vi "Convert Pressure (inHg) to Altitude (ft).vi"(10 "Altimeter Setting (inHg)":dbl=29.9213, 11 "Pressure (inHg)":dbl) -> (3 "Altitude (ft)":dbl)   [LabVIEW 2020, in "LPS Barometric Pressure Sensor.lvclass"]
doc: "Converts pressure in mbar to altitude in meters, using 1976 US Standard Atmosphere model (only applicable up to height of 11km/36,000ft). If altimeter setting (QNH, barometric pressure adjusted to sea level) is given, this function returns an indicated altitude compensated for actual regional pressure; otherwise, it returns the pressure altitude above the standard pressure level of 1013.25mbar or 29.9213 inHg."
uses:
  LPS Barometric Pressure Sensor.lvclass
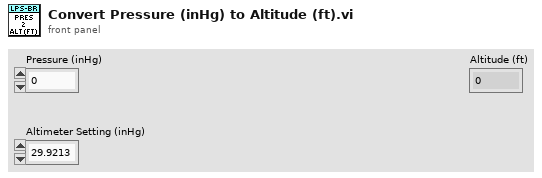
[diagram p1: front panel]
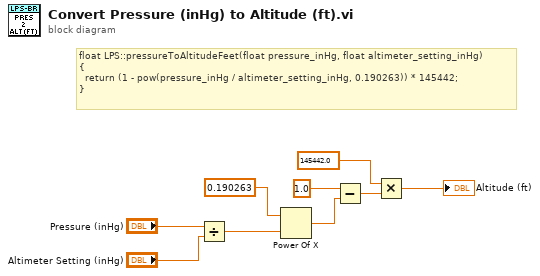
[diagram p0: block diagram]
diagram:
  # "float LPS::pressureToAltitudeFeet(float pressure_inHg, float altimeter_setting_inHg)\n{\n  return (1 - pow(pressure_inHg / altimeter_setting_inHg, 0.190263)) * 145442;\n}"
  n1 = Divide(x="Pressure (inHg)", y="Altimeter Setting (inHg)") -> (x/y=w6:dbl)
  n2 = Power Of X(1:w6, 2:0.190263 ("x")) -> (0:w4:dbl)
  n3 = Subtract(x=1.0, y=w4) -> (x-y=w3:dbl)
  n4 = Multiply(x=145442.0, y=w3) -> (x*y=→"Altitude (ft)":dbl)
